vi "Polynome FID.vi"() -> ()   [LabVIEW 2020, in "ABB-EL3000.lvlib" / "FID.lvlib" / "FID Kalibrierung.lvlib"]
uses:
  FID Kalibrierung.lvlib
  Allgemeine VI/FGV Uras26 Aktion.ctl
  Allgemeine VI/Allgemeine VI.lvlib
  Allgemein/allgemeine Sub-VIs.lvlib
panel:
  in  "Aktiv":bool[](array[boolean])
  in  "Polynomkoeffizienten":sgl[][](array[numeric])
  in  "Abbrechen":bool
  in  "Speichern":bool
  # "THC"
  # "MB1"
  # "MB2"
  # "MB3"
  # "CH4"
  # "Polynomkoeffizienten FID"
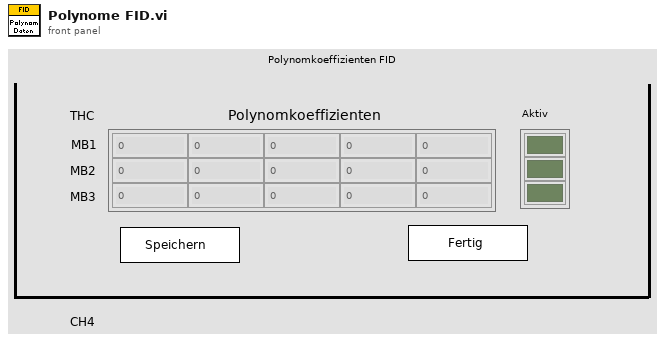
[diagram p1: front panel]
types:
  T1 = typedef "ABB-EL3000.lvlib/Allgemeine VI.lvlib/FGV Uras26 Aktion.ctl" = enum16{"lesen", "CAL-Daten laden", "Messen", "Kalibrieren vorbereiten", "Kalibrieren", "CAL-Daten speichern", "Toleranz schreiben", "CAL-Daten kopieren"}
  T2 = typedef "ABB-EL3000.lvlib/Allgemeine VI.lvlib/FGV Uras26 Aktion.ctl" = enum16{"lesen", "CAL-Daten laden", "Messen", "Kalibrieren vorbereiten", "Kalibrieren", "CAL-Daten speichern", "Toleranz schreiben", "CAL-Daten kopieren", "Polynom", "LIN aktiv", "Polynom Daten speichern", "Rohwert vor Lin", "Rohwert nach Lin"}
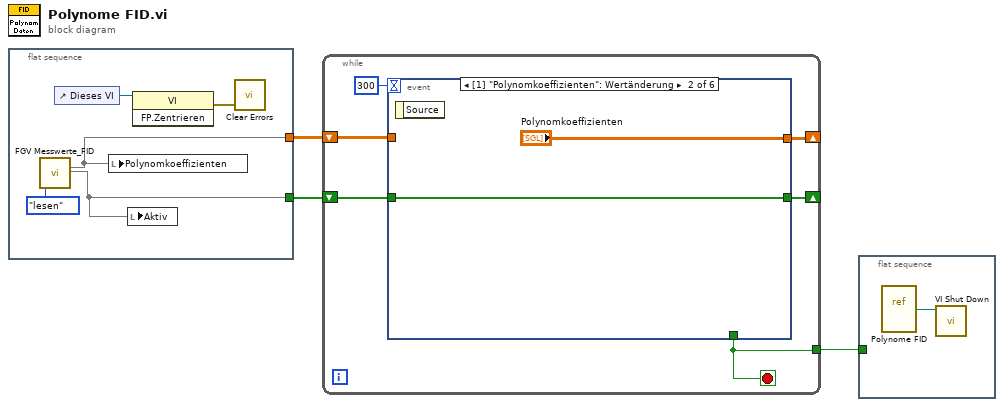
[diagram p0: block diagram]
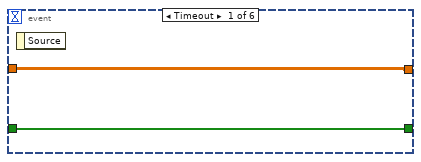
[diagram p2: hidden frame]
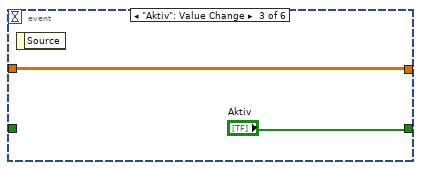
[diagram p3: hidden frame]
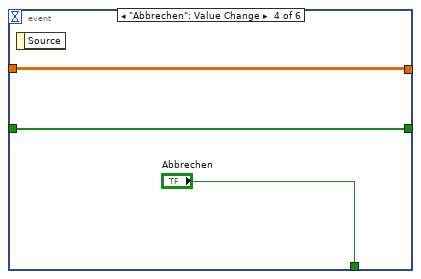
[diagram p4: hidden frame]
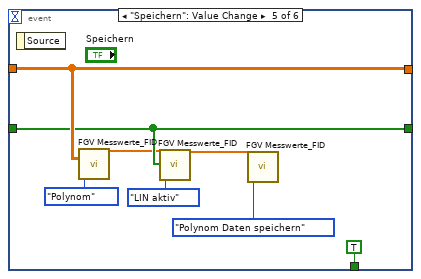
[diagram p5: hidden frame]
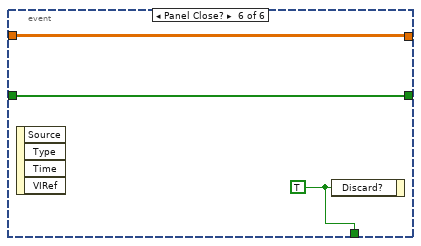
[diagram p6: hidden frame]
diagram:
  n1 = flat-sequence {
    tunnel: [w7] -> w1
    tunnel: [w6] -> w2
    frame #0 {
      n2 = call "FGV Messwerte_FID.vi"("Aktion"=FGV_Uras26_Aktion."lesen") -> (22:w7, 23:w6)  [unwired: 17 in, 8 out]
      n3 = control-ref of="Dieses VI"() -> (w5:refnum<vi>)
      n4 = local write "Polynomkoeffizienten"(w7) -> ()
      n5 = local write "Aktiv"(w6) -> ()
      n6 = invoke class="VI" method="FP.Zentrieren"(reference=w5) -> (error out=w4:errorcluster)  [unwired: 2 in, 2 out]
      n7 = call <vilib>:"Clear Errors.vi"("error in (no error)"=w4) -> ()  [unwired: 5 in, 2 out]
    }
  }
  n8 = while {
    shift-right: [w12] -> _
    shift-left: w1 -> [w13]
    shift-right: [w10] -> _
    shift-left: w2 -> [w11]
    tunnel: [w9] -> w3
    stop <- w9 stop-if-true
    n9 = event shown="[1] \"Polynomkoeffizienten\": Wertänderung" {
      selector: _ -> [_ _ _ _ _ _]
      dyn-events: _ -> [_ _ _ _ _ _]
      timeout: 300 -> [_ _ _ _ _ _]
      tunnel: w13 -> [w16 _ w20 w23 w30 w32]
      tunnel: [w16 "Polynomkoeffizienten" w20 w23 w30 w32] -> w12
      tunnel: w11 -> [w15 w18 _ w22 w28 w33]
      tunnel: [w15 w18 "Aktiv" w22 w28 w33] -> w10
      tunnel: [_ _ _ "Abbrechen" TRUE ("Verwerfen?") w34] -> w9
      event Timeout {
        n10 = event-data() -> ()  [unwired: 1 in, 1 out]
      }
      event "Polynomkoeffizienten": Value Change {
        n11 = event-data() -> ()  [unwired: 1 in, 1 out]
      }
      event "Aktiv": Value Change {
        n12 = event-data() -> ()  [unwired: 1 in, 1 out]
      }
      event "Abbrechen": Value Change {
        n13 = event-data() -> ()  [unwired: 1 in, 1 out]
      }
      event "Speichern": Value Change {
        n14 = event-data() -> ()  [unwired: 1 in, 1 out]
        n15 = call "FGV Messwerte_FID.vi"(2:w30, "Aktion"=FGV_Uras26_Aktion."Polynom") -> ("GasValue"=w27:sgl[])  [unwired: 18 in, 7 out]
        n16 = call "FGV Messwerte_FID.vi"("GasValue"=w27, 3:w28, "Aktion"=FGV_Uras26_Aktion."LIN aktiv") -> ("GasValue"=w25:sgl[])  [unwired: 17 in, 7 out]
        n17 = call "FGV Messwerte_FID.vi"("GasValue"=w25, "Aktion"=FGV_Uras26_Aktion."Polynom Daten speichern") -> ()  [unwired: 18 in, 8 out]
      }
      event Panel Close? {
        w34 = TRUE ("Verwerfen?")
        n18 = event-data() -> ()  [unwired: 1 in, 4 out]
        n19 = event-data("Discard?"=w34) -> ()  [unwired: 1 in, 1 out]
      }
    }
  }
  n20 = flat-sequence {
    tunnel: w3 -> [_]
    frame #0 {
      n21 = vi-ref "Polynome FID.vi"() -> (w35:refnum<vi>)
      n22 = call "VI Shut Down.vi"("VI Referenz"=w35) -> ()  [unwired: 11 in]
    }
  }
